vi "Substitution Degrees.vi"(10 "actual theta":dbl, 11 "cluster":cluster{"velocity":dbl, "target theta":dbl}) -> (3 "output cluster":cluster{"velocity":dbl, "travel angle":dbl})   [LabVIEW 2020]
uses:
  <vilib>/Analysis/coordinate.llb/Angle Range (Degree).ctl
  <vilib>/Analysis/coordinate.llb/Angle Units.ctl
  <vilib>/Analysis/coordinate.llb/Wrap Angle (scalar).vi
  <vilib>/Analysis/NI_AAL_Angle.lvlib
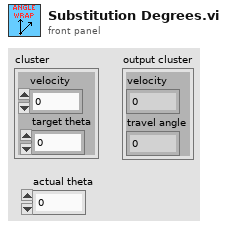
[diagram p1: front panel]
types:
  T1 = typedef "NI_AAL_Angle.lvlib/Angle Units.ctl" = i32
  T2 = typedef "NI_AAL_Angle.lvlib/Angle Range (Degree).ctl" = u16
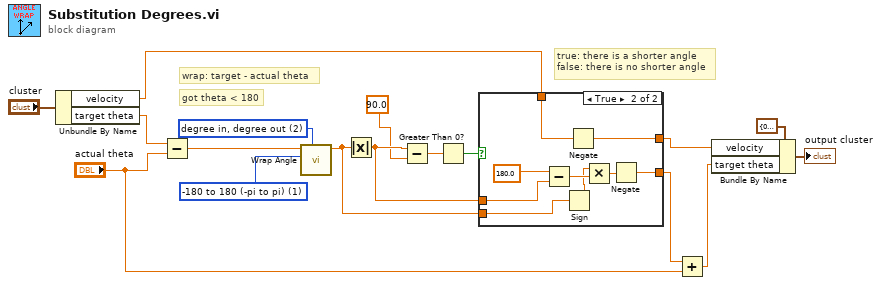
[diagram p0: block diagram]
diagram:
  w16 = T1 2 items=["radian in, radian out", "radian in, degree out", "degree in, degree out", "degree in, radian out"] ("angle units")
  w17 = T2 1 items=["none", "-180 to 180 (-pi to pi)", "0 to 360 (0 to 2pi)"] ("angle range")
  # "true: there is a shorter angle\nfalse: there is no shorter angle"
  # "got theta < 180"
  # "wrap: target - actual theta"
  n1 = Unbundle By Name("cluster") -> ("velocity"=w11:dbl, "target theta"=w14:dbl)
  n2 = Subtract(x=w14, y="actual theta") -> (x-y=w13:dbl)
  n3 = call-poly <vilib>:"Wrap Angle.vi"("angle units"=w16, "angle range"=w17, "angle in"=w13) -> ("angle out"=w5:dbl)  [unwired: 7 in, 1 out]
  n4 = Absolute Value(x=w5) -> (abs(x)=w6:dbl)
  n5 = Subtract(x=w6, y=90.0) -> (x-y=w10:dbl)
  n6 = Greater Than 0?(x=w10) -> (x > 0?=w12:bool)
  n7 = case shown="True" w12 {
    tunnel: w11 -> [w19 w28]
    tunnel: [w19 w27] -> w9
    tunnel: w6 -> [_ w25]
    tunnel: [w18 w26] -> w3
    tunnel: w5 -> [w18 w22]
    frame False {
    }
    frame True {
      n8 = Subtract(x=180.0, y=w25) -> (x-y=w23:dbl)
      n9 = Sign(1:w22) -> (0:w21:dbl)
      n10 = Negate(x=w28) -> (-x=w27:dbl)
      n11 = Multiply(x=w21, y=w23) -> (x*y=w24:dbl)
      n12 = Negate(x=w24) -> (-x=w26:dbl)
    }
  }
  n13 = Add(x=w3, y="actual theta") -> (x+y=w2:dbl)
  n14 = Bundle By Name(cluster=cluster{"velocity":dbl, "target theta":dbl} {"velocity"=0.0, "target theta"=0.0}, "velocity"=w9, "target theta"=w2) -> (→"output cluster":cluster{"velocity":dbl, "target theta":dbl})
